vi "nove_horas.vi"() -> ()   [LabVIEW 2018]
panel:
  out "Variant":variant
  out "String":string
  in  "Listbox":i32(listbox)
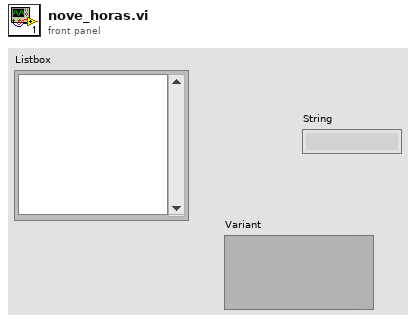
[diagram p1: front panel]
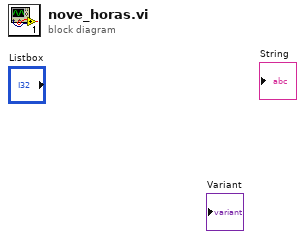
[diagram p0: block diagram]
diagram:
